vi "FestoCPX.vi"() -> ()   [LabVIEW 2016]
uses:
  FestoCPX.Data.ctl
  FestoCPX.Data.Status.ctl
  FestoCPX.State.ctl
  FestoCPX.Data.Sets.ctl
  FestoCPX.DI.Sets.ctl
  FestoCPX.DI.ctl
  FestoCPX.DO.Sets.ctl
  FestoCPX.DO.ctl
  FestoCPX.Action.ctl
  tools/CitTemplate/citTemplate.errData.ctl
  tools/EventLog/EventLog.EventSource.ctl
  Global/ApplicationGlobal.vi
  FestoCPX.Global.vi
  FestoCPX.DI.Signal.ctl
  FestoCPX.DO.Signal.ctl
panel:
  out "error.action":string
  out "error":errorcluster
  out "action":T1
  out "Data":T2={"Status"={"State"=enum."First", "Conn"=refnum, "TS"=timestamp(0 s since 1904-01-01)}, "Sets"={"IP"="", "Timeout_ms"=1, "ReconnectPeriod_s"=0, "Config.DI"=[], "Config.DO"=[]}}
  out "_loop":i32(ring)=4
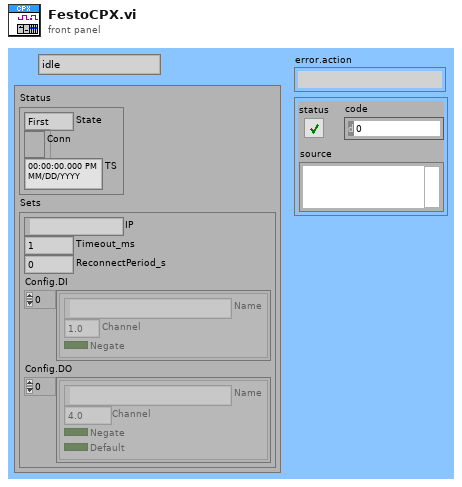
[diagram p1: front panel]
types:
  T1 = typedef "FestoCPX.Action.ctl" = enum32{"idle", "constructor", "destructor", "--- FestoCPX ---", "Init"}
  T2 = typedef "FestoCPX.Data.ctl" = cluster{"Status":T3, "Sets":T5}
  T3 = typedef "FestoCPX.Data.Status.ctl" = cluster{"State":T4, "Conn":refnum<k5>, "TS":timestamp}
  T4 = typedef "FestoCPX.State.ctl" = enum16{"First", "Error", "Init", "Run"}
  T5 = typedef "FestoCPX.Data.Sets.ctl" = cluster{"IP":string, "Timeout_ms":i32, "ReconnectPeriod_s":i32, "Config.DI":T6[], "Config.DO":T8[]}
  T6 = typedef "FestoCPX.DI.Sets.ctl" = cluster{"Name":string, "Channel":T7, "Negate":bool}
  T7 = typedef "FestoCPX.DI.ctl" = enum16{"0.0", "0.1", "0.2", "0.3", "0.4", "0.5", "0.6", "0.7", "1.0", "1.1", "1.2", "1.3", "1.4", "1.5", "1.6", "1.7", "2.0", "2.1", "2.2", "2.3", "2.4", "2.5", "2.6", "2.7", "3.0", "3.1", "3.2", "3.3", "3.4", "3.5", "3.6", "3.7", "4.0", "4.1", "4.2", "4.3", "4.4", "4.5", "4.6", "4.7"}
  T8 = typedef "FestoCPX.DO.Sets.ctl" = cluster{"Name":string, "Channel":T9, "Negate":bool, "Default":bool}
  T9 = typedef "FestoCPX.DO.ctl" = enum16{"4.0", "4.1", "4.2", "4.3", "4.4", "4.5", "4.6", "4.7", "5.0", "5.1", "5.2", "5.3", "5.4", "5.5", "5.6", "5.7", "6.0", "6.1", "6.2", "6.3", "6.4", "6.5", "6.6", "6.7", "Q1K1", "Q1K2", "Q2K1", "Q2K2", "Q3K1", "Q3K2", "Q4K1", "Q4K2", "Q5K1", "Q5K2", "Q6K1", "Q6K2"}
  T10 = typedef "citTemplate.errData.ctl" = cluster{"ts":timestamp, "src":T11, "instance":i32, "action":string, "error":errorcluster, "unconfirmed":bool}
  T11 = typedef "EventLog.EventSource.ctl" = enum16{"All", "Gui", "Ref", "File", "Arch", "Seq", "CPX", "DB", "Laser", "Scan.P", "Scan.O"}
  T12 = typedef "citTemplate.notifierHandle.ctl" = refnum<notifier>
  T13 = typedef "FestoCPX.DO.Signal.ctl" = enum16{"Safety Reset", "Air Main Valve", "Door Lock", "Button LED Start", "Button LED Stop", "Button LED Control", "Traffic LED Red", "Traffic LED Orange", "Traffic LED Green", "Horn", "Laser Interlock", "Laser Trigger", "Laser Fume Extractor", "Product Suction Gripper Slot 1 A", "Product Suction Gripper Slot 1 B", "Product Suction Gripper Slot 2 A", "Product Suction Gripper Slot 2 B", "Product Suction Gripper Slot 3 A", "Product Suction Gripper Slot 3 B", "Product Suction Gripper Slot 4 A", "Product Suction Gripper Slot 4 B", "Product Suction Gripper Final A", "Product Suction Gripper Final B", "Lamp", "Q1 Product Move Work", "Q1 Product Move Home", "Q2 Table Turn Work", "Q2 Table Turn Home", "Q3 Product Lift A", "Q3 Product Lift B", "Q4 Product Arm OK", "Q4 Product Arm NOK", "Q5 Product Arm Work", "Q6 Product BlowOut A", "Q6 Product BlowOut B"}
  T14 = typedef "FestoCPX.DI.Signal.ctl" = enum16{"S.C. Emergency Stop", "S.C. Side Door Close", "S.C. Front Door Close", "S.C. Front Door Secured", "Button Start", "Button Stop", "Button Control", "Product Move Home", "Product Move Work", "Table Position", "Table Lock", "Product Lift A Home", "Product Lift B Home", "Product Arm OK", "Product Arm NOK", "Product Arm Work", "Revolver ID 1", "Revolver ID 2", "Revolver ID 3", "Revolver ID 4", "Revolver ID 5", "Air Pressure Inside", "Air Pressure Inlet", "Product Slot 1 A Present", "Product Slot 1 B Present", "Product Slot 2 A Present", "Product Slot 2 B Present", "Product Slot 3 A Present", "Product Slot 3 B Present", "Product Slot 4 A Present", "Product Slot 4 B Present", "Product Final A Present", "Product Final B Present", "Product Output A Present", "Product Output B Present", "Product Container OK Present", "Product Container NOK Present", "Fork ID 1", "Fork ID 2"}
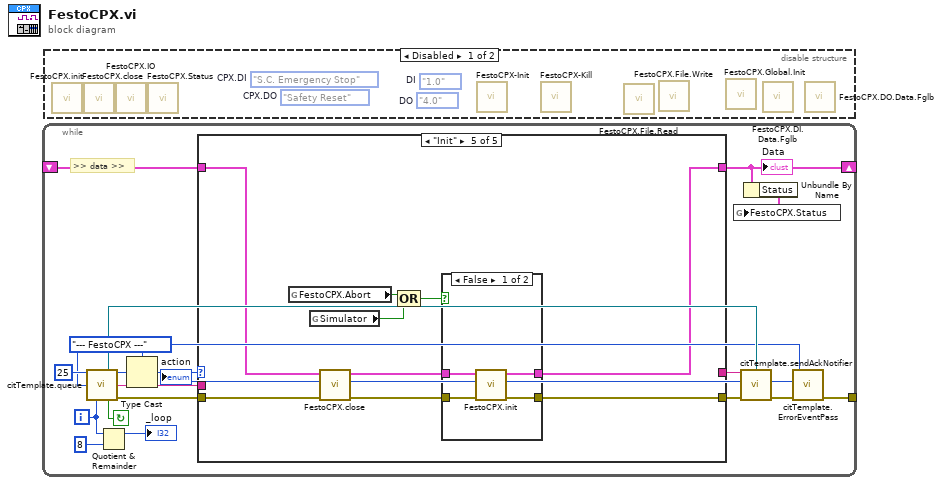
[diagram p0: block diagram]
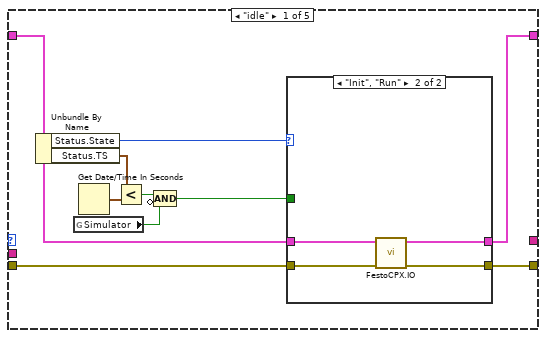
[diagram p3: hidden frame]
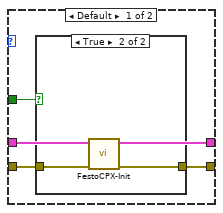
[diagram p4: hidden frame]
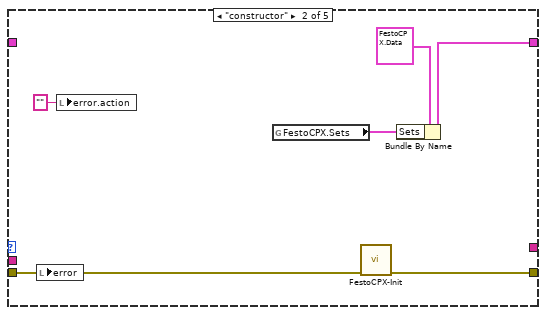
[diagram p6: hidden frame]
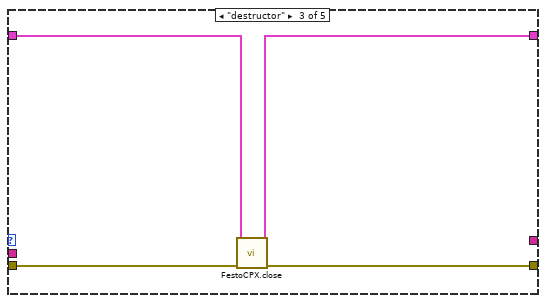
[diagram p7: hidden frame]
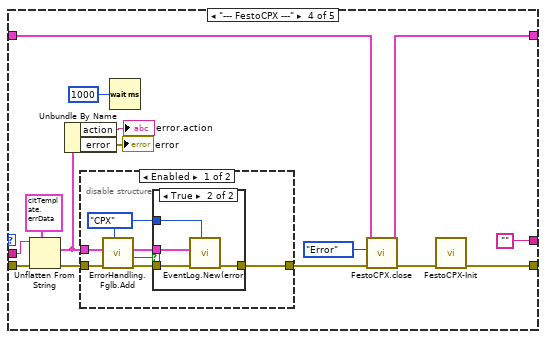
[diagram p8: hidden frame]
diagram:
  n1 = while {
    shift-right: [w2] -> _
    shift-left: _ -> [w13]
    tunnel: [w3] -> _
    i -> [w10]
    stop <- w15 continue-if-true
    w7 = FestoCPX.Action."--- FestoCPX ---" ("states")
    # ">> data >>"
    n2 = call "citTemplate.queue.vi"("ms timeout (250 ms)"=25, "event enum"=w7, "iteration (-1)"=w10) -> ("notifierHandle out"=w12:T12, "event out"=w16:u32, "(flatten) data out"=w14:string, "continue"=w15:bool, "error out"=w11:errorcluster)  [unwired: 2 in, 6 out]
    n3 = Quotient & Remainder(x=w10, y=8) -> (x-y*floor(x/y)=→"_loop":i32)  [unwired: 1 out]
    n4 = Type Cast(type=w7, x=w16) -> (*(type *) &x=w6:T1)
    "action" <- w6
    n5 = case shown="\"Init\"" w6 {
      tunnel: w14 -> [_ _ _ w61 _]
      tunnel: [w26 w40 w47 w58 w84] -> w5
      tunnel: w13 -> [w24 _ w46 w52 w82]
      tunnel: [_ _ _ "" _] -> w4
      tunnel: [w25 w43 w45 w50 w83] -> w2
      tunnel: w11 -> [w27 w39 w48 w60 w81]
      frame "idle" {
        n6 = Unbundle By Name(w24) -> ("Status.State"=w23:T4, "Status.TS"=w19:timestamp)
        n7 = global read "ApplicationGlobal.vi" "Simulator"() -> (w20:bool)
        n8 = Get Date/Time In Seconds() -> (seconds since 1Jan1904=w22:timestamp)
        n9 = Less?(x=w19, y=w22) -> (x < y?=w21:bool)
        n10 = Compound Arithmetic op=AND(w21, invert w20) -> (w18:bool)
        n11 = case shown="\"Init\", \"Run\"" w23 {
          tunnel: w27 -> [w29 w35]
          tunnel: [w28 w36] -> w26
          tunnel: [w31 w37] -> w25
          tunnel: w24 -> [w31 w38]
          tunnel: w18 -> [w30 _]
          frame Default {
            n12 = case shown="True" w30 {
              tunnel: [w32 w33] -> w28
              tunnel: w29 -> [w32 w34]
              frame False {
              }
              frame True {
                n13 = call "FestoCPX-Init.vi"("error in (no error)"=w34) -> ("error out"=w33:errorcluster)  [unwired: 10 in]
              }
            }
          }
          frame "Init", "Run" {
            n14 = call "FestoCPX.IO.vi"("error in"=w35, "Data in"=w38) -> ("error out"=w36:errorcluster, "Data out"=w37:T2)  [unwired: 8 in]
          }
        }
      }
      frame "constructor" {
        n15 = local write "error"(w39) -> ()
        n16 = local write "error.action"("" ("error.action")) -> ()
        n17 = global read "FestoCPX.Global.vi" "FestoCPX.Sets"() -> (w41:T5)
        n18 = call "FestoCPX-Init.vi"("error in (no error)"=w39) -> ("error out"=w40:errorcluster)  [unwired: 10 in]
        n19 = Bundle By Name(cluster=T2 {"Status"={"State"=enum."First", "Conn"=refnum, "TS"=timestamp(0 s since 1904-01-01)}, "Sets"={"IP"="", "Timeout_ms"=0, "ReconnectPeriod_s"=0, "Config.DI"=[], "Config.DO"=[]}} ("Data"), "Sets"=w41) -> (w43:T2)
      }
      frame "destructor" {
        n20 = call "FestoCPX.close.vi"("error in (no error)"=w48, "Data in"=w46) -> ("error out"=w47:errorcluster, "Data out"=w45:T2)  [unwired: 8 in]
      }
      frame "--- FestoCPX ---" {
        n21 = Unflatten From String(type=T10 {"ts"=timestamp(0 s since 1904-01-01), "src"=enum."All", "instance"=0, "action"="", "error"={"status"=FALSE, "code"=0, "source"=""}, "unconfirmed"=FALSE} ("ErrData"), binary string=w61, error in (no error)=w60) -> (value=w56:T10, error out=w57:errorcluster)  [unwired: 2 in, 1 out]
        n22 = Unbundle By Name(w56) -> ("action"=→"error.action":string, "error"=→"error":errorcluster)
        n23 = disable-structure shown="Enabled" {
          disable-tunnel: w57 -> [w68 w75]
          disable-tunnel: w56 -> [w66 _]
          disable-tunnel: [w65 w75] -> w53
          frame Enabled {
            w67 = EventLog.EventSource."CPX" ("Event source")
            n24 = call "ErrorHandling.Fglb.Add.vi"("Event source"=w67, "error in (no error)"=w68, "Error in"=w66) -> ("error out"=w69:errorcluster, "changed?"=w64:bool)  [unwired: 7 in]
            n25 = case shown="True" w64 {
              tunnel: w69 -> [w70 w74]
              tunnel: w67 -> [_ w73]
              tunnel: w66 -> [_ w72]
              tunnel: [w70 w71] -> w65
              frame False {
              }
              frame True {
                n26 = call "EventLog.New(error).vi"("Source (All)"=w73, "error in"=w74, "ErrData"=w72) -> ("error out"=w71:errorcluster)  [unwired: 8 in]
              }
            }
          }
          frame Disabled {
          }
        }
        n27 = Wait (ms)(milliseconds to wait=u32 1000) -> ()  [unwired: 1 out]
        n28 = call "FestoCPX.close.vi"("error in (no error)"=w53, "State (Off)"=FestoCPX.State."Error" ("State @ close"), "Data in"=w52) -> ("error out"=w49:errorcluster, "Data out"=w50:T2)  [unwired: 7 in]
        n29 = call "FestoCPX-Init.vi"("error in (no error)"=w49) -> ("error out"=w58:errorcluster)  [unwired: 10 in]
      }
      frame "Init" {
        n30 = global read "FestoCPX.Global.vi" "FestoCPX.Abort"() -> (w78:bool)
        n31 = global read "ApplicationGlobal.vi" "Simulator"() -> (w76:bool)
        n32 = call "FestoCPX.close.vi"("error in (no error)"=w81, "Data in"=w82) -> ("error out"=w80:errorcluster, "Data out"=w79:T2)  [unwired: 8 in]
        n33 = Compound Arithmetic op=OR(w78, w76) -> (w77:bool)
        n34 = case shown="False" w77 {
          tunnel: [w85 w89] -> w84
          tunnel: w80 -> [w88 w89]
          tunnel: w79 -> [w87 w90]
          tunnel: [w86 w90] -> w83
          frame False {
            n35 = call "FestoCPX.init.vi"("error in (no error)"=w88, "Data in"=w87) -> ("error out"=w85:errorcluster, "Data out"=w86:T2)  [unwired: 8 in]
          }
          frame True {
          }
        }
      }
    }
    "Data" <- w2
    n36 = call "citTemplate.sendAckNotifier.vi"("notification data"=w4, "notifierHandle in"=w12, "error in"=w5) -> ()  [unwired: 13 out]
    n37 = Unbundle By Name(w2) -> ("Status"=w1:T3)
    n38 = global write "FestoCPX.Global.vi" "FestoCPX.Status"(w1) -> ()
    n39 = call "citTemplate.ErrorEventPass.vi"("error in"=w5, "action of error"=w6, "event in"=w7) -> ("error out"=w3:errorcluster)  [unwired: 8 in]
  }
  n40 = disable-structure shown="Disabled" {
    frame Disabled {
      (unwired) FestoCPX.DO."4.0"  # DO
      (unwired) FestoCPX.DI."1.0"  # DI
      (unwired) FestoCPX.DO.Signal."Safety Reset"  # CPX.DO
      (unwired) FestoCPX.DI.Signal."S.C. Emergency Stop"  # CPX.DI
      n41 = call "FestoCPX.init.vi"() -> ()  [unwired: 10 in, 2 out]
      n42 = call "FestoCPX.close.vi"() -> ()  [unwired: 10 in, 2 out]
      n43 = call "FestoCPX.IO.vi"() -> ()  [unwired: 10 in, 2 out]
      n44 = call "FestoCPX.Status.vi"() -> ()  [unwired: 10 in, 2 out]
      n45 = call "FestoCPX-Init.vi"() -> ()  [unwired: 11 in, 1 out]
      n46 = call "FestoCPX-Kill.vi"() -> ()  [unwired: 11 in, 1 out]
      n47 = call "FestoCPX.File.Read.vi"() -> ()  [unwired: 11 in, 1 out]
      n48 = call "FestoCPX.File.Write.vi"() -> ()  [unwired: 11 in, 1 out]
      n49 = call "FestoCPX.Global.Init.vi"() -> ()  [unwired: 11 in, 1 out]
      n50 = call "FestoCPX.DI.Data.Fglb.vi"() -> ()  [unwired: 7 in, 5 out]
      n51 = call "FestoCPX.DO.Data.Fglb.vi"() -> ()  [unwired: 9 in, 3 out]
    }
    frame Enabled {
    }
  }
